vi "Theory Astar FPGAorig.vi"() -> ()   [LabVIEW 2014]
panel:
  out "Main y":i32[](array[numeric])
  out "Main X":i32[](array[numeric])
  out "Y Dest":i32
  out "X dest":i32
  in  "Destination Y":i16
  in  "Destination X":i16
  in  "Start Y":i16
  in  "Start X":i16
  in  "occupancy grid":bool[](array[boolean])=[FALSE, FALSE, FALSE, FALSE, FALSE, FALSE, FALSE, FALSE, FALSE, FALSE, FALSE, FALSE, FALSE, FALSE, FALSE, FALSE, FALSE, FALSE, FALSE, FALSE, FALSE, FALSE, FALSE, FALSE, FALSE, FALSE, FALSE, FALSE, FALSE, FALSE, FALSE, FALSE, FALSE, FALSE, FALSE, FALSE, FALSE, FALSE, FALSE, FALSE, FALSE, FALSE, FALSE, FALSE, FALSE, FALSE, FALSE, FALSE, FALSE, FALSE, FALSE, FALSE, FALSE, FALSE, FALSE, FALSE, FALSE, FALSE, FALSE, FALSE, FALSE, FALSE, FALSE, FALSE, FALSE, FALSE, FALSE, FALSE, FALSE, FALSE, FALSE, FALSE, FALSE, FALSE, FALSE, FALSE, FALSE, FALSE, FALSE, FALSE]
  # "x"
  # "y"
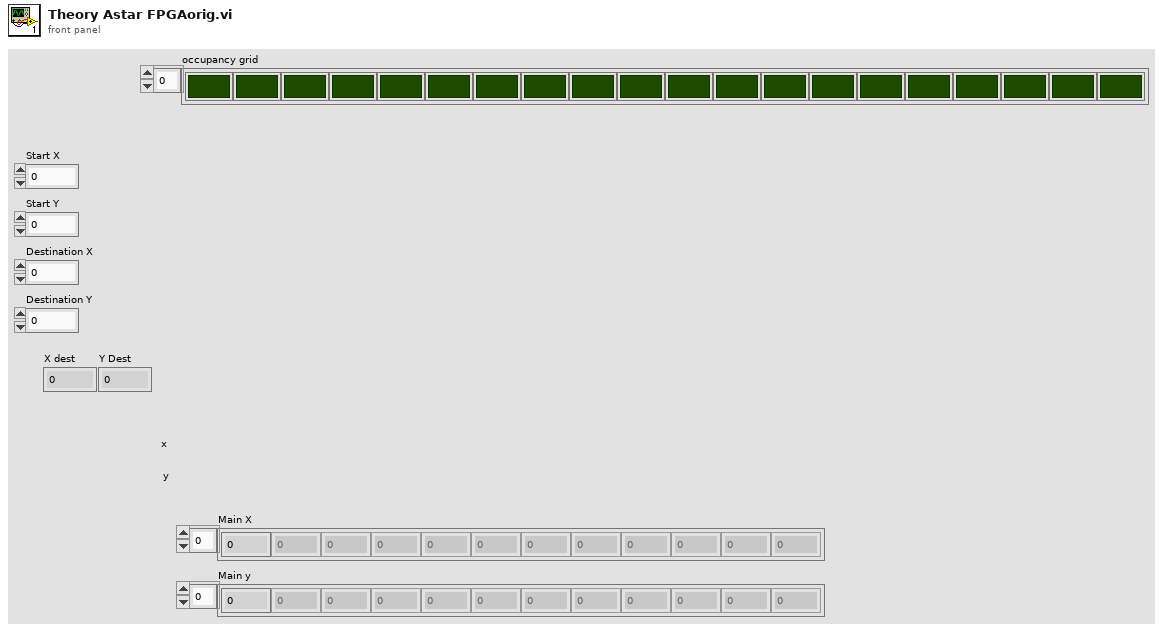
[diagram p1: front panel]
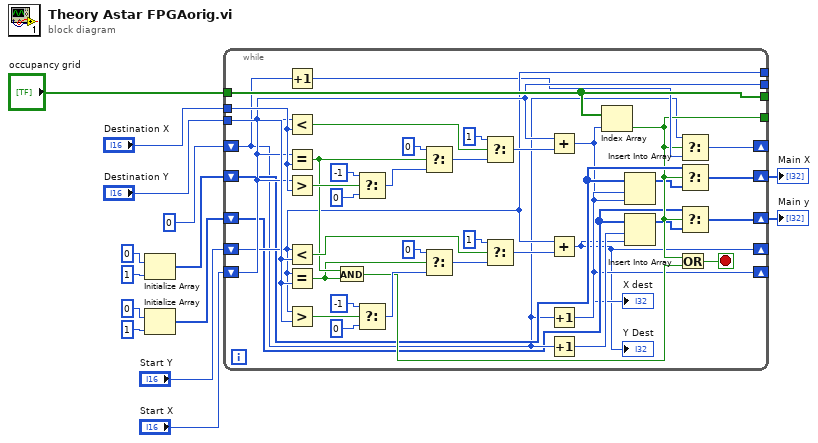
[diagram p0: block diagram]
diagram:
  n1 = Initialize Array(0 ("dimension size"), 1 ("dimension size")) -> (w7:i32[])
  n2 = Initialize Array(0 ("dimension size"), 1 ("dimension size")) -> (w3:i32[])
  n3 = while {
    tunnel: "occupancy grid" -> [w31]
    tunnel: "Destination Y" -> [w55]
    tunnel: "Destination X" -> [w54]
    shift-right: [w16] -> _
    shift-left: "Start X" -> [w30]
    shift-right: [w15] -> _
    shift-left: "Start Y" -> [w29]
    shift-right: [w26] -> w6
    shift-left: w7 -> [w24]
    shift-right: [w27] -> _
    shift-left: 0 -> [w21]
    tunnel: [w31] -> _
    tunnel: [w30] -> _
    tunnel: [w29] -> _
    tunnel: [w22] -> _
    shift-right: [w23] -> w2
    shift-left: w3 -> [w20]
    stop <- w33 stop-if-true
    n4 = Increment(x=w21) -> (x+1=w28:i32)
    n5 = Less?(x=w30, y=w54) -> (x < y?=w46:bool)
    n6 = Equal?(x=w30, y=w54) -> (x = y?=w35:bool)
    n7 = Greater?(x=w30, y=w54) -> (0:w53:bool)
    n8 = Less?(x=w29, y=w55) -> (x < y?=w39:bool)
    n9 = Equal?(x=w29, y=w55) -> (x = y?=w34:bool)
    n10 = Greater?(x=w29, y=w55) -> (0:w38:bool)
    n11 = And(x=w35, y=w34) -> (x .and. y?=w32:bool)
    n12 = Select(t=-1, s=w53, f=0) -> (s? t:f=w49:i32)
    n13 = Select(t=-1, s=w38, f=0) -> (s? t:f=w42:i32)
    n14 = Select(t=0, s=w35, f=w49) -> (s? t:f=w47:i32)
    n15 = Select(t=0, s=w34, f=w42) -> (s? t:f=w40:i32)
    n16 = Select(t=1, s=w46, f=w47) -> (s? t:f=w37:i32)
    n17 = Select(t=1, s=w39, f=w40) -> (s? t:f=w36:i32)
    n18 = Add(x=w30, y=w37) -> (x+y=w16:i32)
    "X dest" <- w16
    n19 = Add(x=w29, y=w36) -> (x+y=w15:i32)
    "Y Dest" <- w15
    n20 = Increment(x=w21) -> (x+1=w25:i32)
    n21 = Increment(x=w21) -> (x+1=w19:i32)
    n22 = Index Array(array=w31, index=w16) -> (element=w22:bool)
    n23 = Insert Into Array(array=w24, index=w25, new element=w16) -> (w18:i32[])
    n24 = Insert Into Array(array=w20, index=w19, new element=w15) -> (w17:i32[])
    n25 = Or(x=w22, y=w32) -> (x .or. y?=w33:bool)
    n26 = Select(t=w21, s=w22, f=w28) -> (s? t:f=w27:i32)
    n27 = Select(t=w24, s=w22, f=w18) -> (s? t:f=w26:i32[])
    n28 = Select(t=w20, s=w22, f=w17) -> (s? t:f=w23:i32[])
  }
  "Main X" <- w6
  "Main y" <- w2
